vi "Existing_Doc.vi"() -> ()   [LabVIEW 2026]
uses:
  <vilib>/Utility/NIReport.llb/Report Type.ctl
  <vilib>/Utility/NIReport.llb/Append Image to Report (path wrap).vi
  <vilib>/Utility/NIReport.llb/NI_report.lvclass
  <vilib>/Utility/NIReport.llb/NI_ReportGenerationCore.lvlib
panel:
  in  "font settings":T1={"Charset (-1)"=-1, "Weight (-1)"=-1, "Name"="", "Size"=" "}
  in  "report type (standard)":T2(ring)=enum."Word"
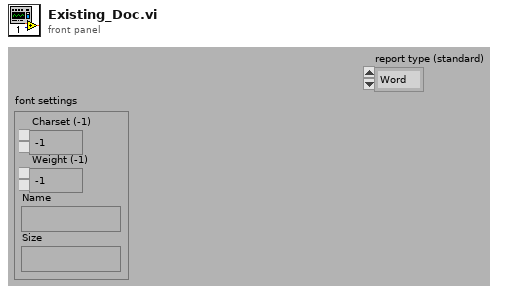
[diagram p1: front panel]
types:
  T1 = cluster{"Charset (-1)":i16, "Weight (-1)":i16, "Name":string, "Size":string}
  T2 = enum16{"Standard Report", "HTML", "Word", "Excel"}
  T3 = typedef "NI_ReportGenerationCore.lvlib/Report Type.ctl" = enum16{"HTML", "Word", "Excel"}
  T4 = cluster{"Italic":enum16{"Italic Unchanged", "Italic On", "Italic Off"}, "Strike Through":enum16{"Strike Through Unchanged", "Strike Through On", "Strike Through Off"}, "Underline":enum16{"Underline Unchanged", "Underline On", "Underline Off"}, "Bold":enum16{"Bold Unchanged", "Bold On", "Bold Off"}}
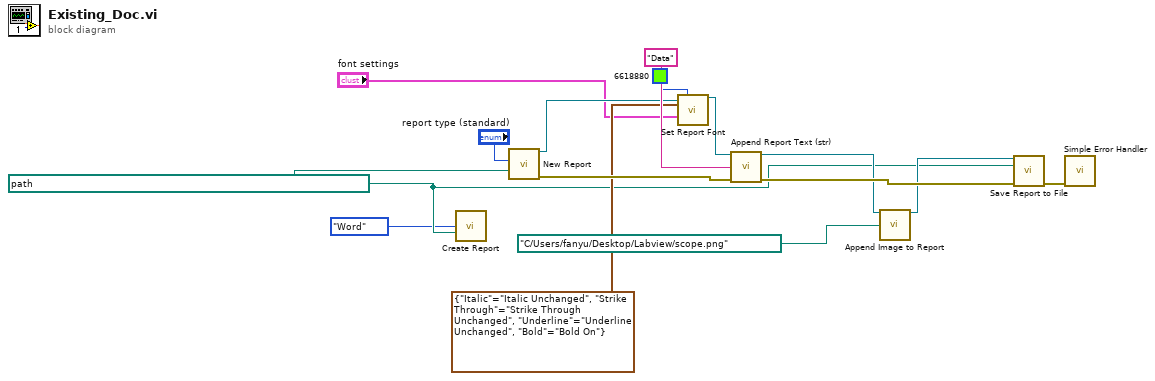
[diagram p0: block diagram]
diagram:
  w2 = path "C:/Users/fanyu/Desktop/Labview/LabVIEW 自動測試報告.docx" ("template (empty)")
  n1 = call <vilib>:"Create Report.vi"("report type"=Report_Type."Word", "template (empty)"=w2) -> ()  [unwired: 12 in, 2 out]
  n2 = call <vilib>:"New Report.vi"("report type"="report type (standard)", "template (empty)"=w2) -> ("report out"=w7:refnum<class "NI_report.lvclass">, "error out"=w11:errorcluster)  [unwired: 12 in]
  n3 = call-dynamic "Set Report Font.vi"("report in"=w7, "text color (unchanged)"=u32 6618880, "text options"=T4 {"Italic"=enum."Italic Unchanged", "Strike Through"=enum."Strike Through Unchanged", "Underline"=enum."Underline Unchanged", "Bold"=enum."Bold On"}, "font settings"="font settings") -> ("report out"=w6:refnum<class "NI_report.lvclass">)  [unwired: 9 in, 2 out]
  n4 = call-dynamic "Append Report Text (str).vi"("report in"=w6, "text"="Data", "error in (no error)"=w11) -> ("report out"=w10:refnum<class "NI_report.lvclass">, "error out"=w14:errorcluster)  [unwired: 9 in, 2 out]
  n5 = call-poly <vilib>:"Append Image to Report.vi"("report in"=w10, "path or URL of image"=path "C:/Users/fanyu/Desktop/Labview/scope.png") -> ("report out"=w8:refnum<class "NI_report.lvclass">)  [unwired: 10 in, 3 out]
  n6 = call-dynamic "Save Report to File.vi"("report in"=w8, "report file path"=w2, "error in (no error)"=w14) -> ("error out"=w13:errorcluster)  [unwired: 11 in, 1 out]
  n7 = call <vilib>:"Simple Error Handler.vi"("error in (no error)"=w13) -> ()  [unwired: 4 in, 5 out]
